vi "Write to APU Report.vi"(7 "report ref":refnum<class "NI_report.lvclass">, 8 "error in":errorcluster, 10 "Report Path":path, 11 "data":T1[](array[typedef])) -> (0 "error out":errorcluster, 3 "report out":refnum<class "NI_report.lvclass">)   [LabVIEW 2018, in "File IO.lvlib"]
uses:
  File IO.lvlib
  Public Controls/Write to Report.ctl
  Public Controls/Report Sheet Names.ctl
  <vilib>/Utility/NIReport.llb/NI_report.lvclass
  <vilib>/Utility/NIReport.llb/Report Type.ctl
  <vilib>/Utility/error.llb/Error Cluster From Error Code.vi
  <vilib>/ErrorRing/Error Ring.xnode
  <vilib>/Utility/NIReport.llb/NI_ReportGenerationCore.lvlib
  <vilib>/Utility/NIReport.llb/Excel/NI_Excel.lvclass
  <vilib>/addons/_office/NI_ReportGenerationToolkit.lvlib
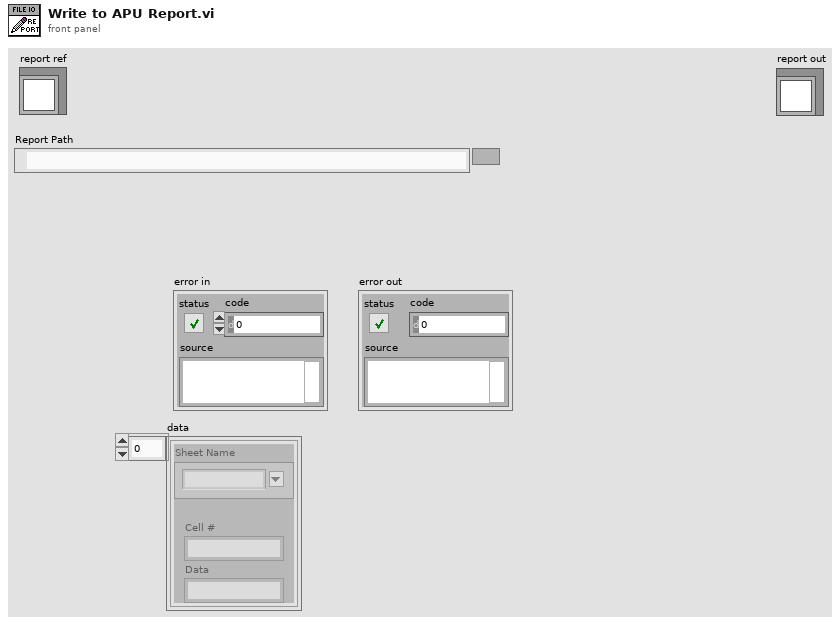
[diagram p1: front panel]
types:
  T1 = typedef "File IO.lvlib/Write to Report.ctl" = cluster{"Sheet Name":T2, "Cell #":string, "Data":string}
  T2 = typedef "File IO.lvlib/Report Sheet Names.ctl" = string
  T3 = typedef "NI_ReportGenerationCore.lvlib/Report Type.ctl" = enum16{"HTML", "Word", "Excel"}
  T4 = enum16{"maximized", "minimized", "normal", "no change"}
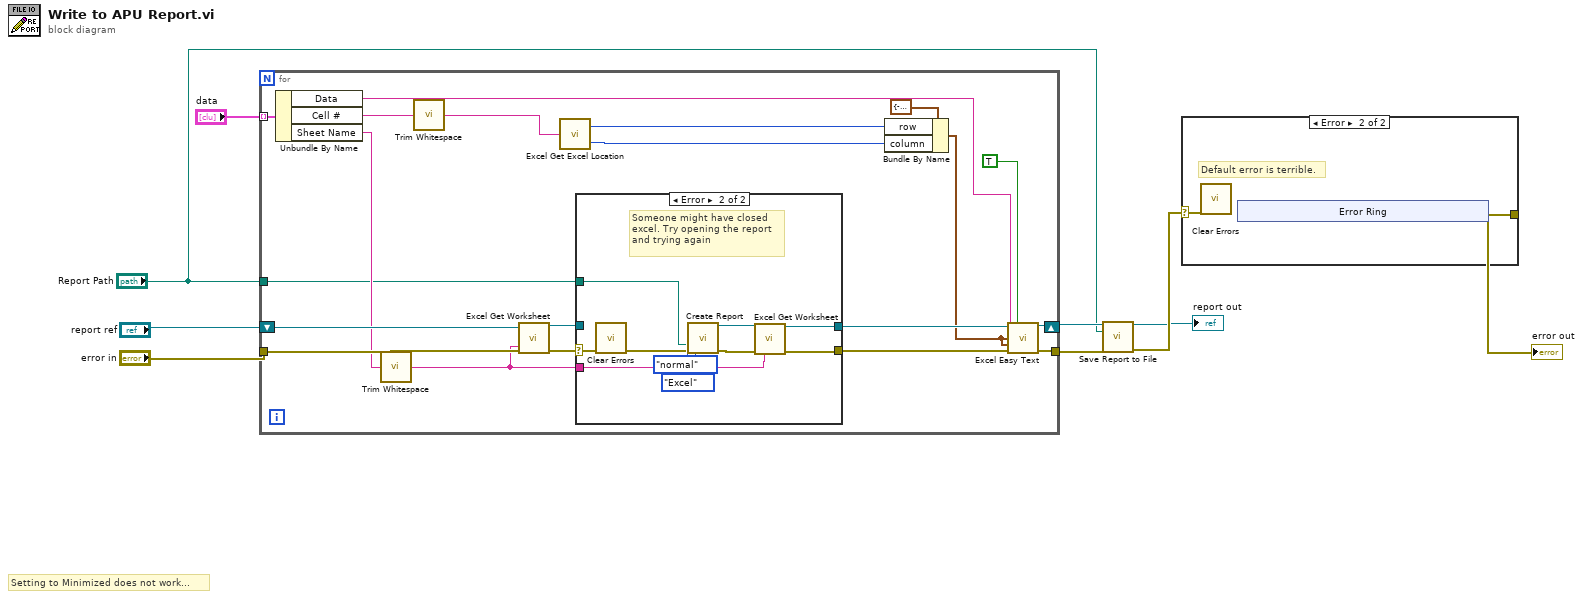
[diagram p0: block diagram]
diagram:
  # "Setting to Minimized does not work..."
  n1 = for {
    tunnel: "data" -> [w17] mode=indexing
    tunnel: "error in" -> [w28]
    tunnel: [w20] -> w4
    shift-right: [w19] -> w5
    shift-left: "report ref" -> [w29]
    tunnel: "Report Path" -> [w12]
    n2 = Unbundle By Name(w17) -> ("Data"=w21:string, "Cell #"=w27:string, "Sheet Name"=w18:T2)
    n3 = call <vilib>:"Trim Whitespace.vi"("string"=w18) -> ("trimmed string"=w14:string)  [unwired: 1 in]
    n4 = call <vilib>:"Trim Whitespace.vi"("string"=w27) -> ("trimmed string"=w15:string)  [unwired: 1 in]
    n5 = call <vilib>:"Excel Get Worksheet.vi"("report in"=w29, "error in (no error)"=w28, "name (\"\")"=w14) -> ("report out"=w10:refnum<class "NI_report.lvclass">, "error out"=w11:errorcluster)  [unwired: 11 in]
    n6 = call <vilib>:"Excel Get Excel Location.vi"("cell's name"=w15) -> ("row"=w25:i32, "column"=w24:i32)
    n7 = case shown="Error" w11 {
      selector: w11 -> [w31 w41]
      tunnel: [w31 w34] -> w23
      tunnel: w12 -> [_ w37]
      tunnel: w14 -> [_ w35]
      tunnel: [w30 w32] -> w22
      tunnel: w10 -> [w30 _]
      frame No Error {
      }
      frame Error {
        # "Someone might have closed\nexcel. Try opening the report\nand trying again"
        n8 = call <vilib>:"Clear Errors.vi"("error in (no error)"=w41) -> ("error out"=w38:errorcluster)  [unwired: 5 in, 1 out]
        n9 = call <vilib>:"Create Report.vi"("window state (normal)"=T4."normal", "report type"=Report_Type."Excel", "template (empty)"=w37, "error in (no error)"=w38) -> ("report out"=w33:refnum<class "NI_report.lvclass">, "error out"=w36:errorcluster)  [unwired: 10 in]
        n10 = call <vilib>:"Excel Get Worksheet.vi"("report in"=w33, "error in (no error)"=w36, "name (\"\")"=w35) -> ("report out"=w32:refnum<class "NI_report.lvclass">, "error out"=w34:errorcluster)  [unwired: 11 in]
      }
    }
    n11 = Bundle By Name(cluster=cluster{"row":i32, "column":i32} {"row"=-1, "column"=-1} ("start (-1, -1)"), "row"=w25, "column"=w24) -> (w16:cluster{"row":i32, "column":i32})
    n12 = call <vilib>:"Excel Easy Text.vi"("report in"=w22, "border? (F)"=TRUE, "text"=w21, "start (-1, -1)"=w16, "end (-1, -1)"=w16, "error in (no error)"=w23) -> ("report out"=w19:refnum<class "NI_report.lvclass">, "error out"=w20:errorcluster)  [unwired: 5 in, 3 out]
  }
  n13 = call-dynamic "Save Report to File.vi"("report in"=w5, "report file path"="Report Path", "error in (no error)"=w4) -> ("report out"=→"report out":refnum<class "NI_report.lvclass">, "error out"=w2:errorcluster)  [unwired: 11 in]
  n14 = case shown="Error" w2 {
    selector: w2 -> [w42 w44]
    tunnel: [w42 w43] -> w7
    frame No Error {
    }
    frame Error {
      # "Default error is terrible."
      n15 = call <vilib>:"Clear Errors.vi"("error in (no error)"=w44) -> ()  [unwired: 5 in, 2 out]
      n16 = xnode "Error Ring"() -> ("error out"=w43:errorcluster)
    }
  }
  "error out" <- w7
